vi "save.vi"(8 "error in (no error)":errorcluster, 10 "operation":T1(ring)=enum."open or create", 11 "Refnum in":refnum<file>) -> (0 "error out":errorcluster, 2 "Recorder State":T2, 3 "Refnum out":refnum<file>)   [LabVIEW 2013]
uses:
  eodrecorderstates.ctl
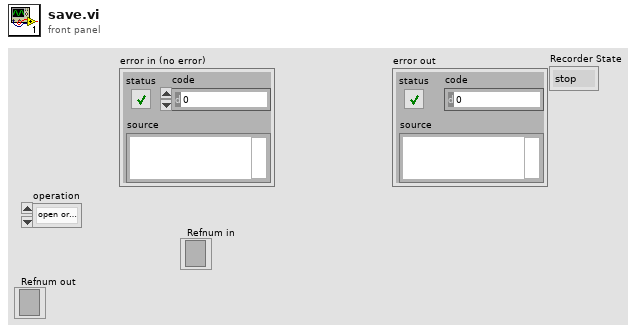
[diagram p1: front panel]
types:
  T1 = enum16{"open", "replace", "create", "open or create", "replace or create", "replace or create with confirmation"}
  T2 = typedef "eodrecorderstates.ctl" = enum16{"stop", "initialize", "live data", "capture data", "analyze data", "open data", "display opened data", "write to file"}
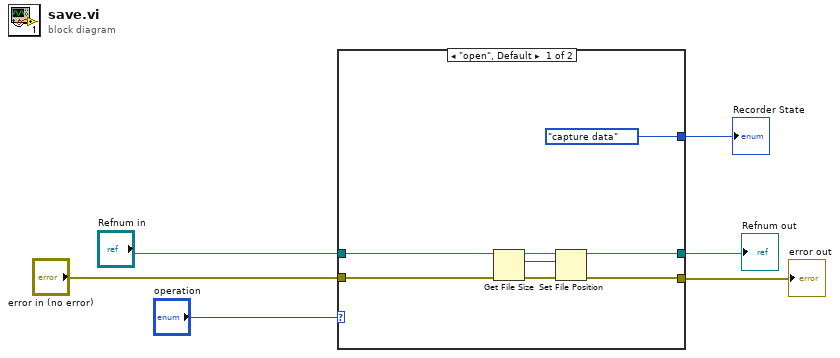
[diagram p0: block diagram]
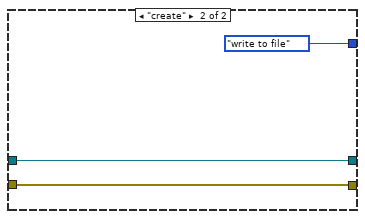
[diagram p2: hidden frame]
diagram:
  n1 = case shown="\"open\", Default" "operation" {
    tunnel: "Refnum in" -> [w8 w17]
    tunnel: "error in (no error)" -> [w9 w16]
    tunnel: [w7 w17] -> w2
    tunnel: [w11 w16] -> w5
    tunnel: [eodrecorderstates."capture data" ("Enum") eodrecorderstates."write to file" ("Enum")] -> w4
    frame "open", Default {
      n2 = Get File Size(file=w8, error in=w9) -> (refnum out=w14:refnum<file>, size (in bytes)=w12:i64, 0:w13:errorcluster)
      n3 = Set File Position(offset (in bytes) (0)=w12, refnum=w14, error in=w13) -> (refnum out=w7:refnum<file>, error out=w11:errorcluster)  [unwired: 1 in]
    }
    frame "create" {
    }
  }
  "error out" <- w5
  "Recorder State" <- w4
  "Refnum out" <- w2
